vi "Start.vi"(8 "error in":errorcluster, 11 "IMAQdx Continuous Acquisition in":refnum<class "IMAQdx Triggered Continuous Acquisition.lvclass">) -> (0 "error out":errorcluster, 3 "IMAQdx Continuous Acquisition out":refnum<class "IMAQdx Triggered Continuous Acquisition.lvclass">)   [LabVIEW 2024, in "IMAQdx Triggered Continuous Acquisition.lvclass"]
uses:
  IMAQdx Triggered Continuous Acquisition.lvclass
  IMAQdx Triggered Continuous Acquisition.lvclass/IMAQdx Triggered Continuous Acquisition.ctl
  <vilib>/vision/driver/NI_Vision_Acquisition_Software.lvlib
  Base/IMAQdx Base Configure Strategy.lvclass
  D:/git/HAL/HAL-Devices/Source/Configure Strategies/IMAQdx Strategies/Base/IMAQdx Base Configure Strategy.lvclass
  D:/git/HAL/Source/Interfaces/IConfigure/IConfigure.lvclass
  D:/git/HAL/Source/Interfaces/IClose/IClose.lvclass
  D:/git/HAL/Source/Interfaces/IInitialize/IInitialize.lvclass
  D:/git/HAL/Source/Interfaces/IValidate Configuration/IValidate Configuration.lvclass
  D:/git/HAL/HAL-Devices/Source/Configure Strategies/IMAQdx Strategies/Continuous Acquisition/IMAQdx Triggered Continuous Acquisition.lvclass
  D:/git/HAL/Source/Interfaces/IRead Image/IRead Images/IRead Image.lvclass
  D:/git/HAL/Source/Interfaces/IRunnable/IRunnable.lvclass
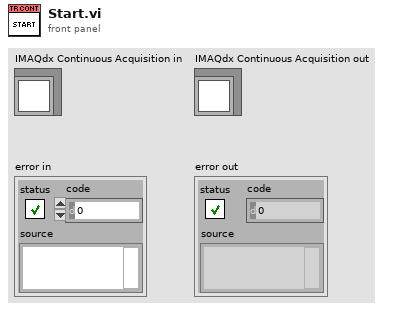
[diagram p1: front panel]
types:
  T1 = typedef "IMAQdx.ctl" = refnum<k21>
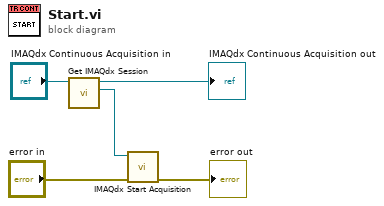
[diagram p0: block diagram]
diagram:
  n1 = call "Get IMAQdx Session.vi"("IMAQdx Base Configure Strategy in"="IMAQdx Continuous Acquisition in") -> ("IMAQdx Session"=w3:T1, "IMAQdx Base Configure Strategy out"=→"IMAQdx Continuous Acquisition out":refnum<class "IMAQdx Triggered Continuous Acquisition.lvclass">)  [unwired: 9 in]
  n2 = call <vilib>:"IMAQdx Start Acquisition.vi"("error in"="error in", "Session In"=w3) -> ("error out"=→"error out":errorcluster)  [unwired: 8 in, 1 out]
